vi "CRUD Testbed2.vi"() -> ()   [LabVIEW 2020]
uses:
  Vehicle/Vehicle.lvclass
  VehicleMap/VehicleMap.lvclass
  C:/Program Files/National Instruments/LabVIEW 2020/vi.lib/Viviota/shared/ORM.lvlibp/ORM/TypeMap/TypeMap.lvclass
  Vehicle2/Vehicle2.lvclass
  <vilib>/Viviota/shared/ORM.lvlibp/Transaction Logger/Log Map/LogMap.lvclass
  <vilib>/Viviota/shared/ORM.lvlibp/ORM/TypeMap/TypeMap.lvclass
  <vilib>/Viviota/shared/ORM_ADONet.lvlibp/ADOMapper/ADOMapper.lvclass
  C:/Program Files/National Instruments/LabVIEW 2020/vi.lib/Viviota/shared/ORM.lvlibp/ORM/SqlMapper/SqlMapper.lvclass
  <vilib>/Viviota/shared/ORM_DBC_Mssql.lvlibp/DBC.lvclass
  C:/Program Files/National Instruments/LabVIEW 2020/vi.lib/Viviota/shared/ORM.lvlibp/ORM/DbConnection/DbConnection.lvclass
  <vilib>/Viviota/shared/ORM_DBC_Npgsql.lvlibp/DBC.lvclass
  <vilib>/Viviota/shared/ORM_Dapper.lvlibp/DapMapper/DapperMapper.lvclass
  <vilib>/Viviota/shared/ORM_DBC_Sqlite.lvlibp/DBC.lvclass
  <vilib>/Viviota/shared/ORM_DBC_Odbc.lvlibp/DBC.lvclass
  Vehicle2/Vehicle2.lvclass/Vehicle2.ctl
  Vehicle2/Write Make.vi
  Vehicle2/Write Model.vi
  Vehicle2/Write Year.vi
  Vehicle2/Write VehicleID.vi
  ca214fdc-7268-4a0d-ad9e-ca0273076739.vi
  46eb3f52-05cf-44df-b166-33ffa5ec5273.vi
  52118b1f-51ce-407b-b922-af4080c0147a.vi
  be60da36-9ccc-4b79-a3b1-32d87cd80171.vi
  2db5b6ec-2611-4d27-a0a2-e5505da9d599.vi
  Vehicle2/Read Make.vi
  Vehicle2/Read Model.vi
  Vehicle2/Read Year.vi
  Vehicle2/Read VehicleID.vi
  ca214fdc-7268-4a0d-ad9e-ca0273076739.vi/35b31214-e0d6-4ae0-b34c-13eba9df70db.vi
  ca214fdc-7268-4a0d-ad9e-ca0273076739.vi/2e8f1eab-5a58-47e6-9224-d0a2895e31fd.vi
  46eb3f52-05cf-44df-b166-33ffa5ec5273.vi/ce8babb2-619c-4b95-b634-e027cd54a13e.vi
  46eb3f52-05cf-44df-b166-33ffa5ec5273.vi/383c36e0-7191-4c70-923d-4cc1411f3794.vi
  46eb3f52-05cf-44df-b166-33ffa5ec5273.vi/dcffdf9a-60b2-440f-af14-9d618c05381d.vi
  52118b1f-51ce-407b-b922-af4080c0147a.vi/bf74eca6-e633-4dc5-891a-edef426d4fd9.vi
  be60da36-9ccc-4b79-a3b1-32d87cd80171.vi/93c2cd5d-a53a-4cc2-b8c3-9c3eef6598b6.vi
  2db5b6ec-2611-4d27-a0a2-e5505da9d599.vi/a9ccc3c9-891a-4d80-8d4f-837bdef88ccd.vi
  2db5b6ec-2611-4d27-a0a2-e5505da9d599.vi/8216614f-f413-45b3-8111-14f8d0271ea5.vi
  2db5b6ec-2611-4d27-a0a2-e5505da9d599.vi/fc6a5c23-d21f-4d2c-895e-66da96fa9491.vi
  2db5b6ec-2611-4d27-a0a2-e5505da9d599.vi/fc6a5c23-d21f-4d2c-895e-66da96fa9491.vi/9d007ba8-e96f-4737-8d8a-6b46cf7f5c4a.vi
  2db5b6ec-2611-4d27-a0a2-e5505da9d599.vi/fc6a5c23-d21f-4d2c-895e-66da96fa9491.vi/050765a8-e5d4-4415-b637-62775228e838.vi
  <vilib>/Viviota/shared/ORM.lvlibp/ORM/TypeMap/Write Table Name.vi
  <vilib>/Viviota/shared/ORM.lvlibp/ORM/TypeMap/Write Autokey.vi
  <vilib>/Viviota/shared/ORM.lvlibp/ORM/TypeMap/Read KeyProperties.vi
  <vilib>/Viviota/shared/ORM.lvlibp/Transaction Logger/Log Map/Write Log Table Name.vi
  <vilib>/Viviota/shared/ORM.lvlibp/Transaction Logger/Log Map/Write IncludeObjRepresentation.vi
  <vilib>/Viviota/shared/ORM.lvlibp/ORM/SqlMapper/Write DbConnection.vi
  <vilib>/Utility/error.llb/Error Cluster From Error Code.vi
  <vilib>/Viviota/shared/ORM.lvlibp/ORM/TypeMap/Read TypeMap.vi
  <vilib>/Viviota/shared/ORM.lvlibp/ORM/SqlMapper/End Transaction.vi
  <vilib>/Viviota/shared/ORM.lvlibp/ORM/TypeMap/Where.vi
  <vilib>/Viviota/shared/ORM.lvlibp/ORM/Query Result/Next.vi
  <vilib>/Viviota/shared/ORM.lvlibp/ORM/TypeMap/ToLabVIEW_Wrap.vi
  <vilib>/Viviota/shared/ORM.lvlibp/ORM/Query Result/Query Result.lvclass
panel:
  out "KeyProperties":string[](array[string])=["Id"]
  in  "Where":string[](array[string])
  out "output cluster":T1(array[cluster])
  out "error out 2":errorcluster
  in  "VehicleCluster":T2
  out "affectedRows":i32
  out "error out":errorcluster
  in  "Enum":T3(ring)
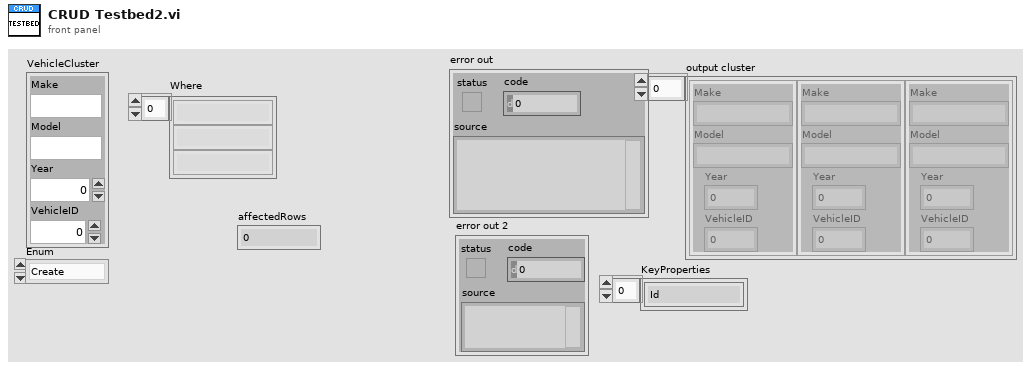
[diagram p1: front panel]
types:
  T1 = cluster{"Make":string, "Model":string, "Year":i32, "VehicleID":u64}[]
  T2 = cluster{"Make":string, "Model":string, "Year":i32, "VehicleID":u64}
  T3 = enum16{"Create", "Read", "Update", "Destroy", "ReadAll"}
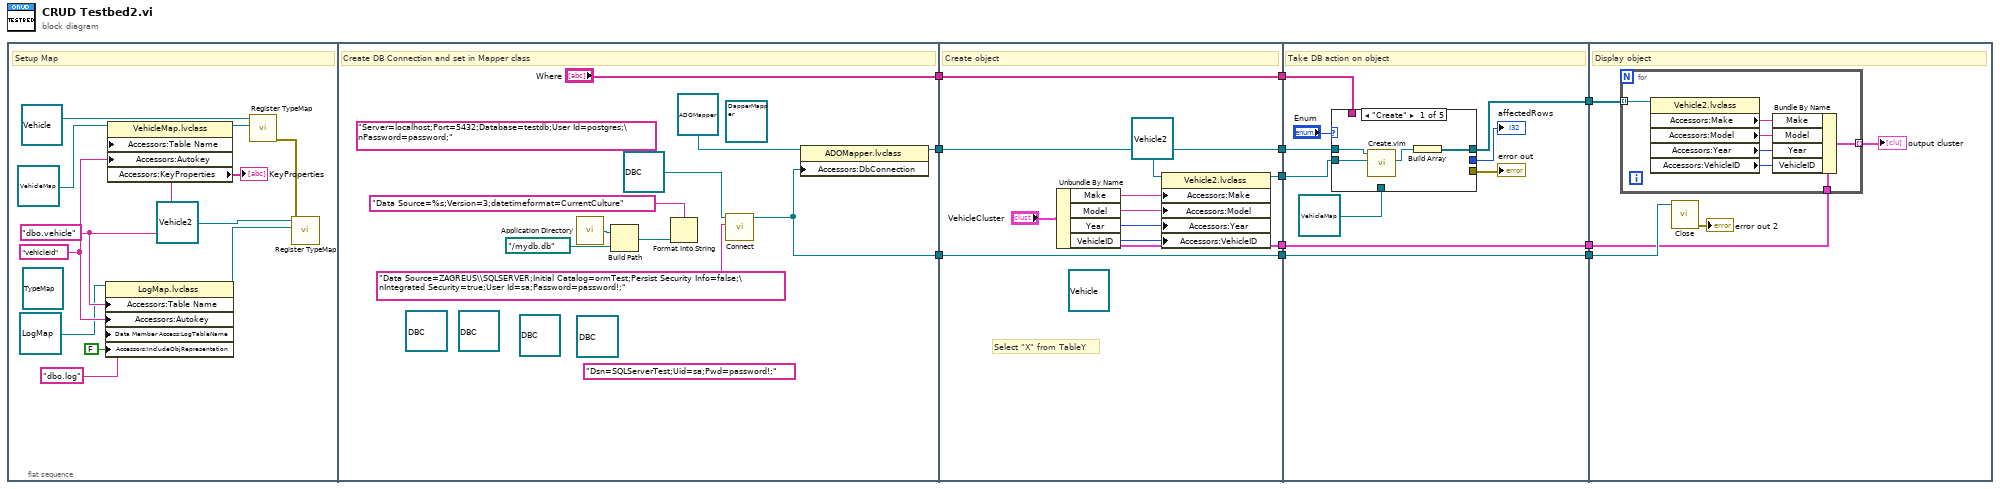
[diagram p0: block diagram]
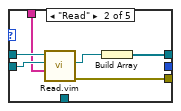
[diagram p2: hidden frame]
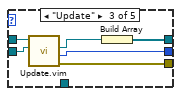
[diagram p3: hidden frame]
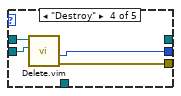
[diagram p4: hidden frame]
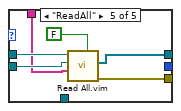
[diagram p5: hidden frame]
diagram:
  n1 = flat-sequence {
    tunnel: [w29] -> w11
    tunnel: [w27] -> w3
    tunnel: ["Where"] -> w1
    tunnel: w11 -> [w42]
    tunnel: ["VehicleCluster"] -> w10
    tunnel: [w43] -> w9
    tunnel: [w42] -> w8
    tunnel: [w37] -> w4
    tunnel: w3 -> [w37]
    tunnel: [w35] -> w2
    tunnel: w1 -> [w35]
    tunnel: w10 -> [w49]
    tunnel: w9 -> [w51]
    tunnel: w8 -> [w50]
    tunnel: [w49] -> w7
    tunnel: [w48] -> w6
    tunnel: [w45] -> w5
    tunnel: w4 -> [w45]
    tunnel: w2 -> [w44]
    tunnel: w7 -> [w80]
    tunnel: w6 -> [w84]
    tunnel: w5 -> [w83]
    frame #0 {
      (unwired) refnum<class "TypeMap.lvclass"> refnum ("TypeMap in")
      w16 = "vehicleid" ("Autokey")
      w17 = "dbo.vehicle" ("Log Table Name")
      # "Setup Map"
      n2 = property class="LogMap.lvclass"(reference=refnum<class "LogMap.lvclass"> refnum ("ORM.lvlibp:LogMap.lvclass"), "Accessors:Table Name"=w17, "Accessors:Autokey"=w16, "Data Member Access:LogTableName"="dbo.log" ("LogTableName"), "Accessors:IncludeObjRepresentation"=FALSE ("IncludeObjRepresentation")) -> (reference out=w18:refnum<class "LogMap.lvclass">)  [unwired: 1 in, 1 out]
      n3 = property class="VehicleMap.lvclass"(reference=refnum<class "VehicleMap.lvclass"> refnum ("VehicleMap.lvclass"), "Accessors:Table Name"=w17, "Accessors:Autokey"=w16) -> (reference out=w21:refnum<class "VehicleMap.lvclass">, "Accessors:KeyProperties"=→"KeyProperties":string[])  [unwired: 1 in, 1 out]
      n4 = call <vilib>:"Register TypeMap.vi"("TypeMap in"=w21, "object in"=refnum<class "Vehicle.lvclass"> refnum ("Vehicle.lvclass")) -> ("error out"=w15:errorcluster)  [unwired: 7 in, 2 out]
      n5 = call <vilib>:"Register TypeMap.vi"("error in (no error)"=w15, "TypeMap in"=w18, "object in"=refnum<class "Vehicle2.lvclass"> refnum ("Vehicle2.lvclass")) -> ()  [unwired: 6 in, 3 out]
    }
    frame #1 {
      (unwired) "Dsn=SQLServerTest;Uid=sa;Pwd=password!;" ("Connection String")
      (unwired) refnum<class "DBC.lvclass"> refnum ("ORM_DBC_Odbc.lvlibp:DBC.lvclass")
      (unwired) refnum<class "DBC.lvclass"> refnum ("SQLConnection Type")
      (unwired) refnum<class "DBC.lvclass"> refnum ("SqliteConnection in")
      (unwired) refnum<class "DapperMapper.lvclass"> refnum ("Dapper.lvlib:DapperMapper.lvclass")
      (unwired) refnum<class "DBC.lvclass"> refnum ("PostgresqlConnection in")
      (unwired) "Server=localhost;Port=5432;Database=testdb;User Id=postgres;\nPassword=password;" ("Connection String")
      # "Create DB Connection and set in Mapper class"
      n6 = call <vilib>:"Application Directory.vi"() -> ("Application Directory"=w32:path)
      n7 = Build Path(base path=w32, name or relative path=path "../mydb.db" ("file out")) -> (appended path=w33:path)
      n8 = Format Into String(format string="Data Source=%s;Version=3;datetimeformat=CurrentCulture" ("connectionStringName"), w33) -> ()  [unwired: 2 in, 2 out]
      n9 = call-dynamic "Connect.vi"("Connection String"="Data Source=ZAGREUS\\SQLSERVER;Initial Catalog=ormTest;Persist Security Info=false;\nIntegrated Security=true;User Id=sa;Password=password!;", "SQLConnection Type"=refnum<class "DBC.lvclass"> refnum) -> ("SQLConnection out"=w27:refnum<class "DBC.lvclass">)  [unwired: 8 in, 1 out]
      n10 = property class="ADOMapper.lvclass"(reference=refnum<class "ADOMapper.lvclass"> refnum ("ADONet.lvlib:ADOMapper.lvclass"), "Accessors:DbConnection"=w27) -> (reference out=w29:refnum<class "ADOMapper.lvclass">)  [unwired: 1 in, 1 out]
    }
    frame #2 {
      (unwired) refnum<class "Vehicle.lvclass"> refnum ("Vehicle.lvclass")
      # "Select \"X\" from TableY"
      # "Create object"
      n11 = Unbundle By Name("VehicleCluster") -> ("Make"=w41:string, "Model"=w40:string, "Year"=w39:i32, "VehicleID"=w36:u64)
      n12 = property class="Vehicle2.lvclass"(reference=refnum<class "Vehicle2.lvclass"> refnum ("Vehicle2.lvclass"), "Accessors:Make"=w41, "Accessors:Model"=w40, "Accessors:Year"=w39, "Accessors:VehicleID"=w36) -> (reference out=w43:refnum<class "Vehicle2.lvclass">)  [unwired: 1 in, 1 out]
    }
    frame #3 {
      # "Take DB action on object"
      n13 = case shown="\"Create\"" "Enum" {
        tunnel: w51 -> [w55 w62 w65 w72 w77]
        tunnel: w50 -> [w56 w63 w69 w73 w79]
        tunnel: [w57 w59 w64 _ w75] -> w48
        tunnel: [_ w60 w66 w71 w78] -> w53
        tunnel: [_ _ w67 w70 _] -> w47
        tunnel: refnum<class "VehicleMap.lvclass"> refnum ("VehicleMap.lvclass") -> [_ _ _ _ _]
        tunnel: w44 -> [_ w58 _ _ w74]
        frame "Create" {
          n14 = call "Create.vim"("object in"=w55, "SqlMapper in"=w56) -> ("object out"=w54:refnum<class "Vehicle2.lvclass">)  [unwired: 6 in, 3 out]
          n15 = Build Array(w54) -> (w57:refnum<class "Vehicle2.lvclass">[])
        }
        frame "Read" {
          n16 = call "Read.vim"("Where"=w58, "object in"=w62, "SqlMapper in"=w63) -> ("error out"=w60:errorcluster, "object out"=w61:refnum<class "Vehicle2.lvclass">)  [unwired: 5 in, 2 out]
          n17 = Build Array(w61) -> (w59:refnum<class "Vehicle2.lvclass">[])
        }
        frame "Update" {
          n18 = call "Update.vim"("object in"=w65, "SqlMapper in"=w69) -> ("error out"=w66:errorcluster, "affectedRows"=w67:i32, "object out"=w68:refnum<class "Vehicle2.lvclass">)  [unwired: 6 in, 1 out]
          n19 = Build Array(w68) -> (w64:refnum<class "Vehicle2.lvclass">[])
        }
        frame "Destroy" {
          n20 = call "Delete.vim"("object in"=w72, "SqlMapper in"=w73) -> ("error out"=w71:errorcluster, "affectedRows"=w70:i32)  [unwired: 7 in, 1 out]
        }
        frame "ReadAll" {
          n21 = call "Read All.vim"("Select All"=FALSE ("Select *"), "WHERE"=w74, "Object"=w77, "SqlMapper in"=w79) -> ("error out"=w78:errorcluster, "Query Results"=w75:refnum<class "Vehicle2.lvclass">[])  [unwired: 5 in, 1 out]
        }
      }
      "error out" <- w53
      "affectedRows" <- w47
    }
    frame #4 {
      # "Display object"
      n22 = for {
        tunnel: w84 -> [w89] mode=indexing
        tunnel: [w86] -> w81 mode=indexing
        tunnel: w80 -> [w85]
        n23 = property class="Vehicle2.lvclass"(reference=w89) -> ("Accessors:Make"=w91:string, "Accessors:Model"=w90:string, "Accessors:Year"=w88:i32, "Accessors:VehicleID"=w87:i32)  [unwired: 1 in, 2 out]
        n24 = Bundle By Name(cluster=w85, "Make"=w91, "Model"=w90, "Year"=w88, "VehicleID"=w87) -> (w86:T2)
      }
      "output cluster" <- w81
      n25 = call-dynamic "Close.vi"("DbConnection in"=w83) -> ("error out"=→"error out 2":errorcluster)  [unwired: 10 in]
    }
  }
